vi "createFolder.vi"(11 "字符串":string) -> ()   [LabVIEW 2011]
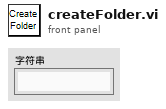
[diagram p1: front panel]
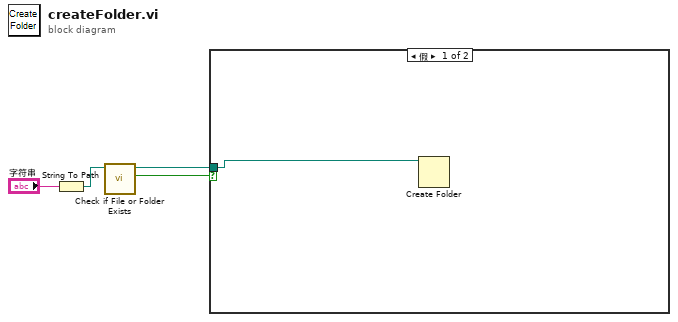
[diagram p0: block diagram]
diagram:
  n1 = String To Path(string="字符串") -> (path=w4:path)
  n2 = call <vilib>:"Check if File or Folder Exists.vi"("path"=w4) -> ("file or folder exists?"=w3:bool, "dup path"=w1:path)  [unwired: 8 in, 1 out]
  n3 = case shown="假" w3 {
    tunnel: w1 -> [w5 _]
    frame False {
      n4 = Create Folder(path (use dialog)=w5) -> ()  [unwired: 2 in, 3 out]
    }
    frame True {
    }
  }
